vi "Read Input buffer size.vi"(8 "error in (no error)":errorcluster, 11 "Spectrum Recorder too in":refnum<class "Spectrum Recorder too.lvclass">) -> (0 "error out":errorcluster, 2 "Input buffer size":i32=8192 format="0x%x (0d%d)", 3 "Spectrum Recorder too out":refnum<class "Spectrum Recorder too.lvclass">)   [LabVIEW 2024, in "Spectrum Recorder too.lvclass"]
uses:
  Spectrum Recorder too.lvclass
  Spectrum Recorder too.lvclass/Spectrum Recorder too.ctl
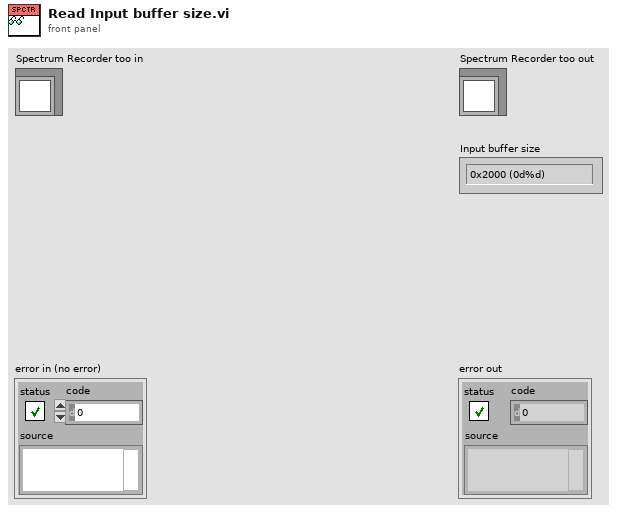
[diagram p1: front panel]
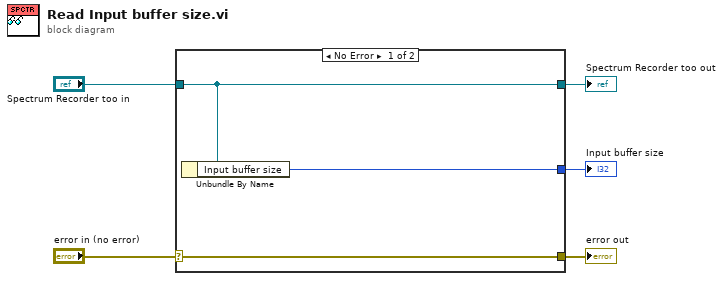
[diagram p0: block diagram]
diagram:
  n1 = case shown="No Error" "error in (no error)" {
    selector: "error in (no error)" -> [w8 w9]
    tunnel: [w8 w9] -> w4
    tunnel: [w7 w10] -> w2
    tunnel: "Spectrum Recorder too in" -> [w7 w10]
    tunnel: [w6 _] -> w1
    frame No Error {
      n2 = Unbundle By Name(w7) -> ("Input buffer size"=w6:i32)
    }
    frame Error {
    }
  }
  "error out" <- w4
  "Spectrum Recorder too out" <- w2
  "Input buffer size" <- w1
